vi "Patrick Builder.vi"() -> ()   [LabVIEW 2019]
uses:
  VIPM/Typedefs/File Type--enum.ctl
  <vilib>/Utility/sysdir.llb/System Directory Type.ctl
  <vilib>/Hampel Software Engineering/Git API/Git API/GIT-api.lvclass
  <vilib>/Utility/file.llb/Read Delimited Spreadsheet (string).vi
  <vilib>/Utility/file.llb/Write Delimited Spreadsheet (string).vi
  <vilib>/JKI/VIPM API/VIPM API_vipm_api.lvlib
  VIPM/VIPM.lvclass
  Git/Git.lvclass
panel:
  out "repository path":path
  out "Latest EXE":path
  out "Latest VIP":path
  in  "Mode":T1
  in  "Create File List":bool
  out "Package Builder":string
  in  "Clear Notes":bool
  in  "Release Notes":string
  in  "Append Notes":bool
  in  "ALL":bool
  in  "Patch +1":bool
  out "Selected File List":string
  in  "Publish":bool
  in  "Open List":bool
  in  "Build":bool
  in  "Preview":bool
  out "Status":string
  in  "File List":i32(listbox)
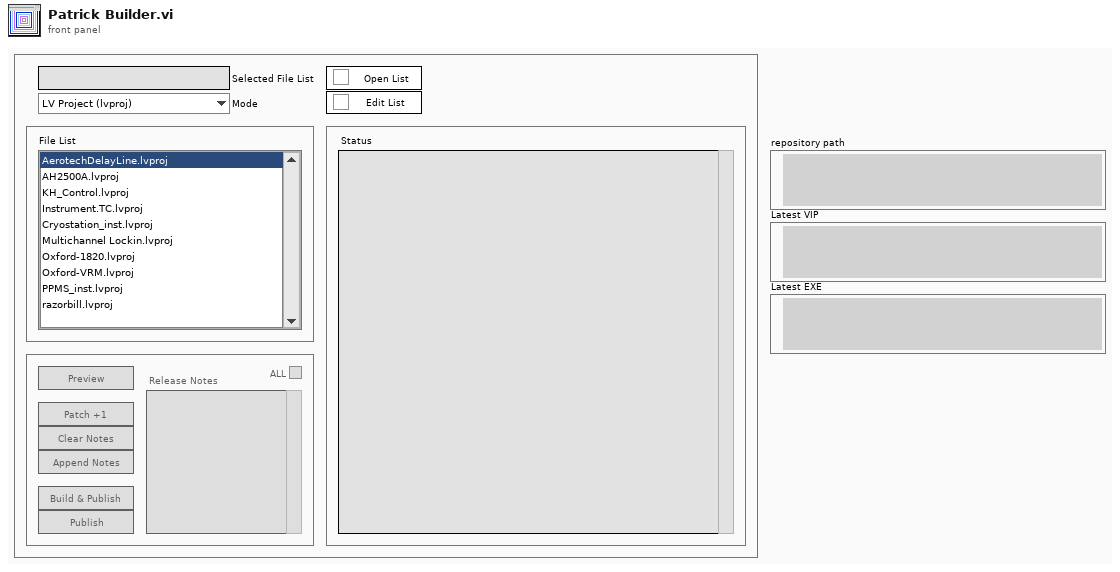
[diagram p1: front panel]
types:
  T1 = typedef "VIPM.lvclass/File Type--enum.ctl" = enum16{"LV Project (lvproj)", "Build Spec (vipb)", "Package (vip)"}
  T2 = enum32{"Invalid", "Standard", "Closed", "Hidden", "Minimized", "Maximized"}
  T3 = enum32{"invalid app kind", "Development System", "Run Time System", "Student Edition", "Embedded LabVIEW", "Evaluation", "Custom"}
  T4 = enum8{"Enabled", "Disabled", "Disabled and Grayed Out"}
  T5 = cluster{"Core":cluster{"Current VI Reference":refnum<vi>, "Close Panel on Exit?":bool}, "lvproj paths":path[], "vipb paths":path[], "vip paths":path[], "selected path":path, "config path":path, "Mode":T1, "git-api":refnum<class "GIT-api.lvclass">}
  T6 = typedef "System Directory Type.ctl" = i32
  T7 = cluster{"Current VI Reference":refnum<vi>, "Close Panel on Exit?":bool}
  T8 = typedef "VIPM API_vipm_api.lvlib/VI Package Build Spec Data Cluster_vipm_api.ctl" = cluster{"Package Version":T9, "Product Name":string, "Company Name":string, "Author Name (Person or Company)":string, "Product Homepage (URL)":string, "Legal Copyright":string, "License Agreement Name":string, "Product Description Summary":string, "Product Description":string, "Release Notes - Change Log":string}
  T9 = typedef "VIPM API_vipm_api.lvlib/Version Info Cluster_vipm_api.ctl" = cluster{"major":u32, "minor":u32, "patch":u32, "build":u32}
  T10 = typedef "VIPM API_vipm_api.lvlib/Repository Info Cluster_vipm_api.ctl" = cluster{"Repository Name":string, "Repository Folder Location":path}
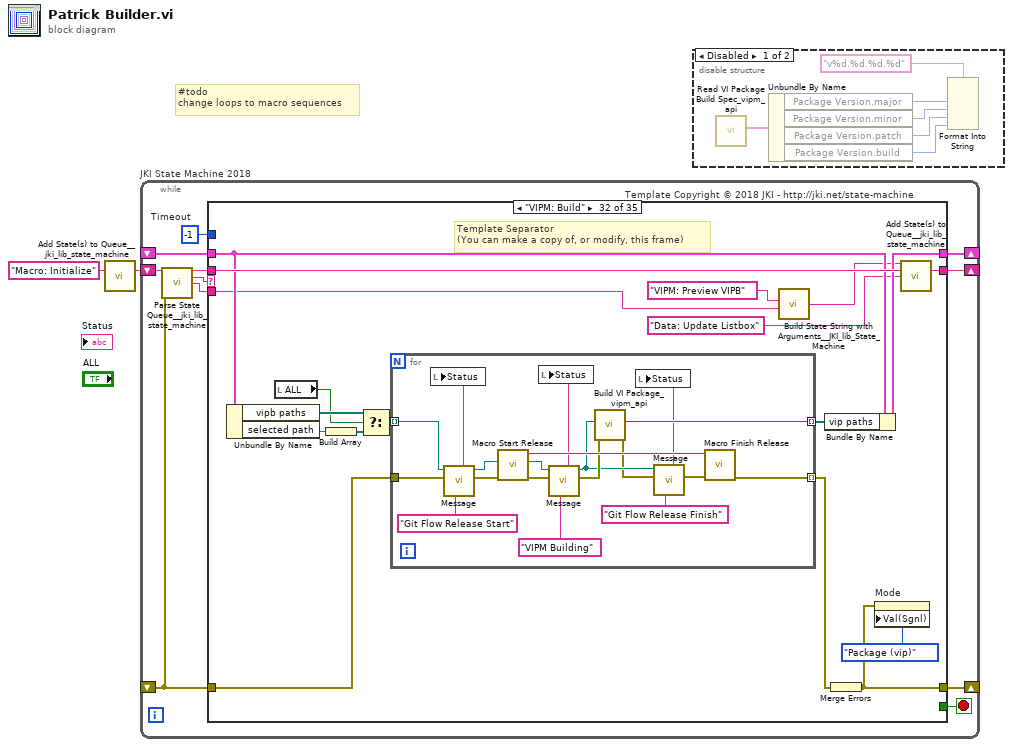
[diagram p0: block diagram]
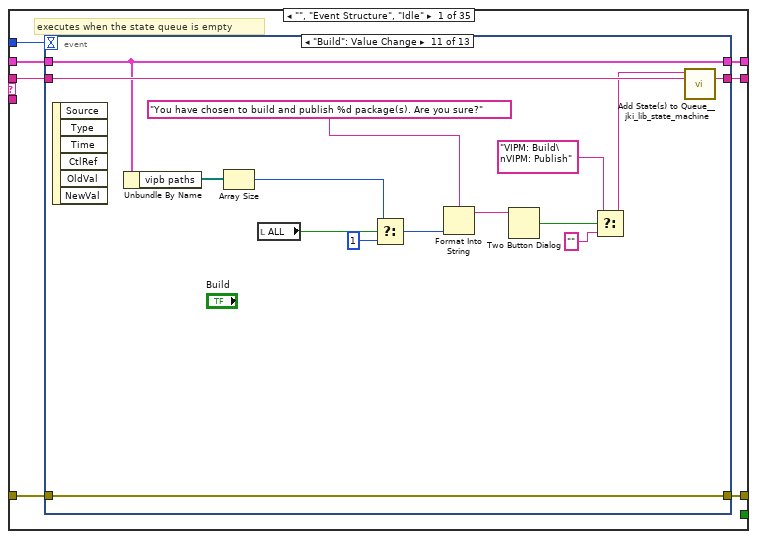
[diagram p3: hidden frame]
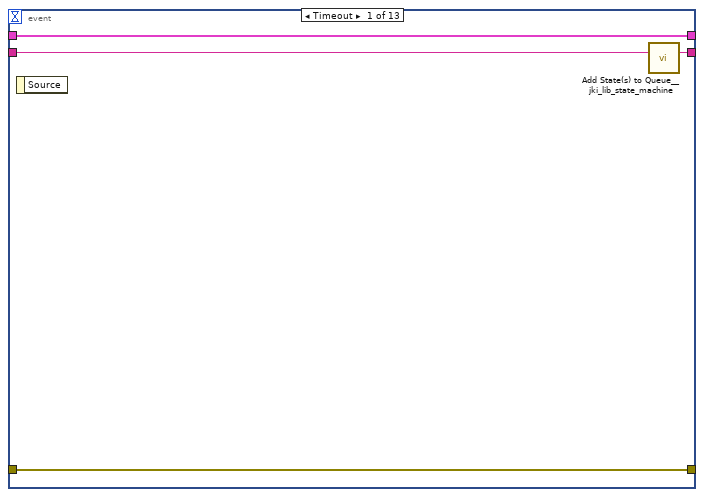
[diagram p4: hidden frame]
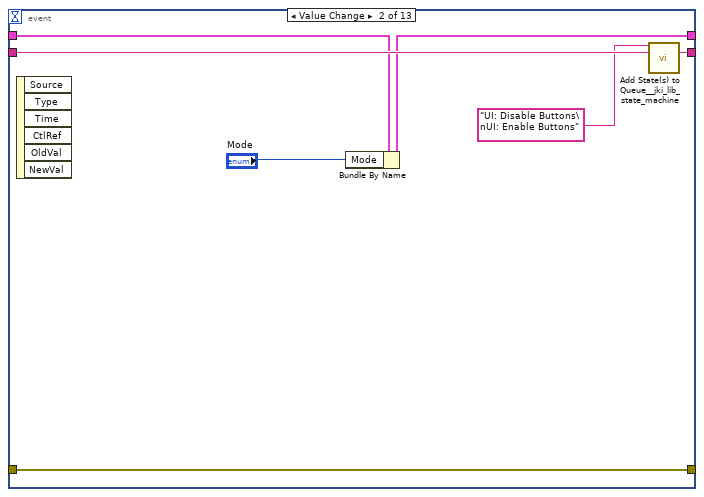
[diagram p5: hidden frame]
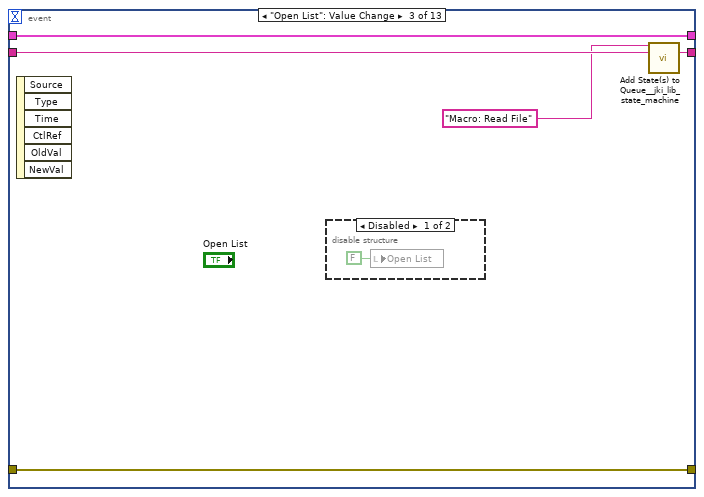
[diagram p6: hidden frame]
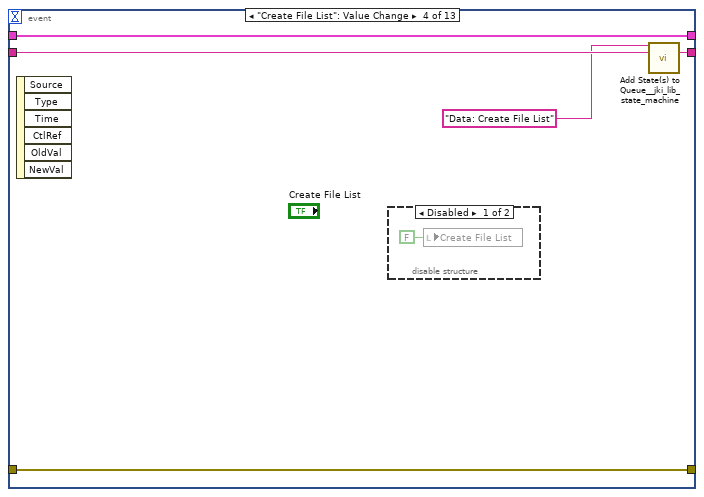
[diagram p8: hidden frame]
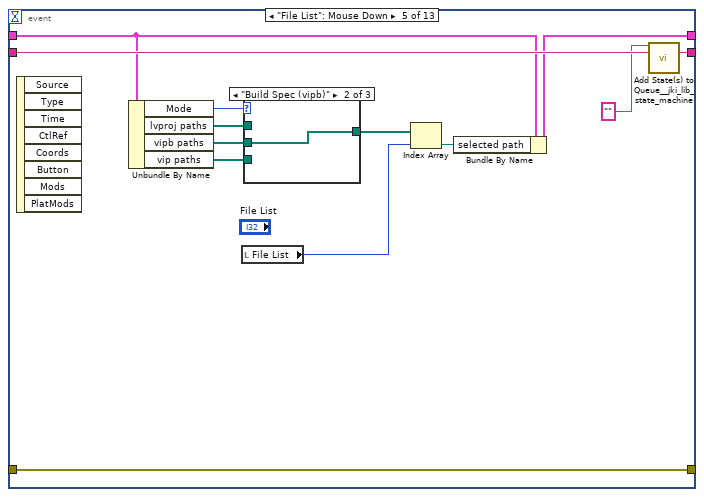
[diagram p10: hidden frame]
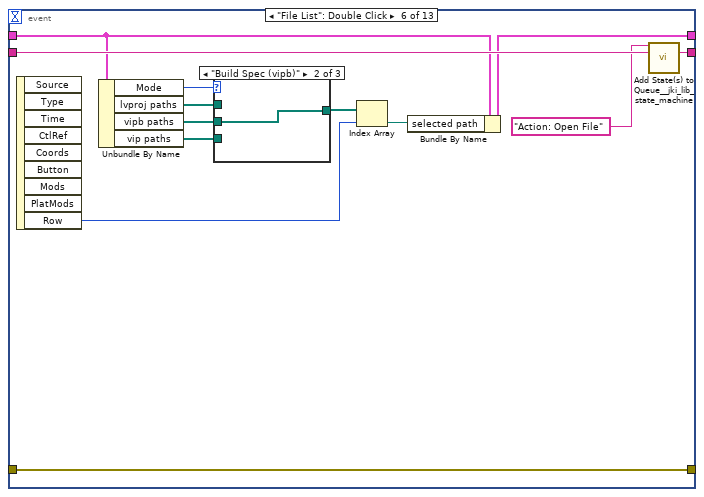
[diagram p13: hidden frame]
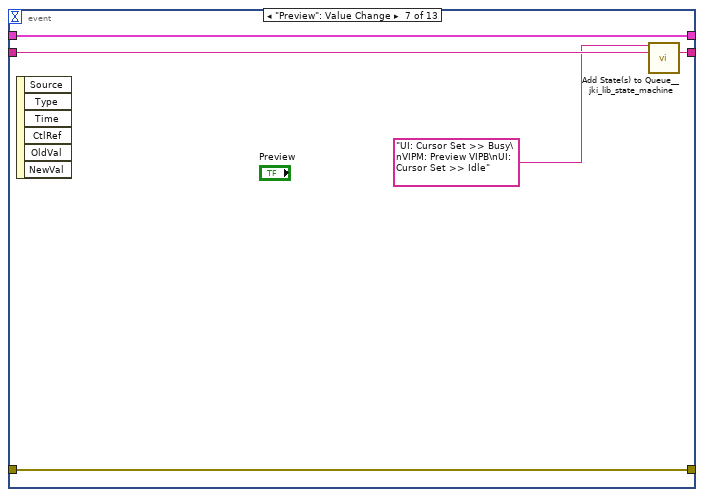
[diagram p16: hidden frame]
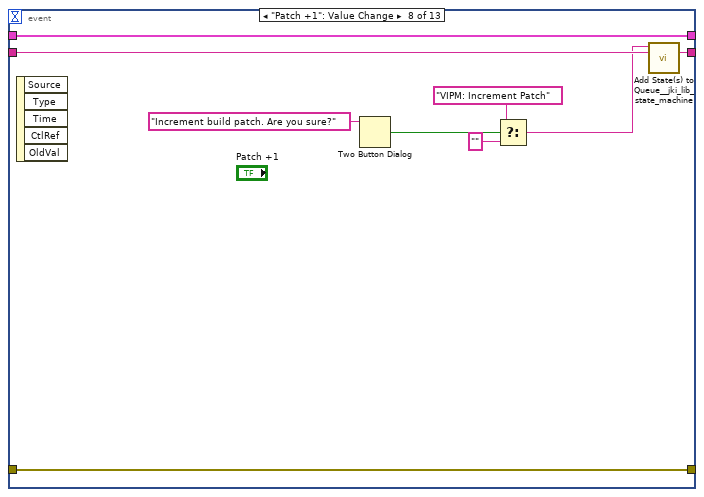
[diagram p17: hidden frame]
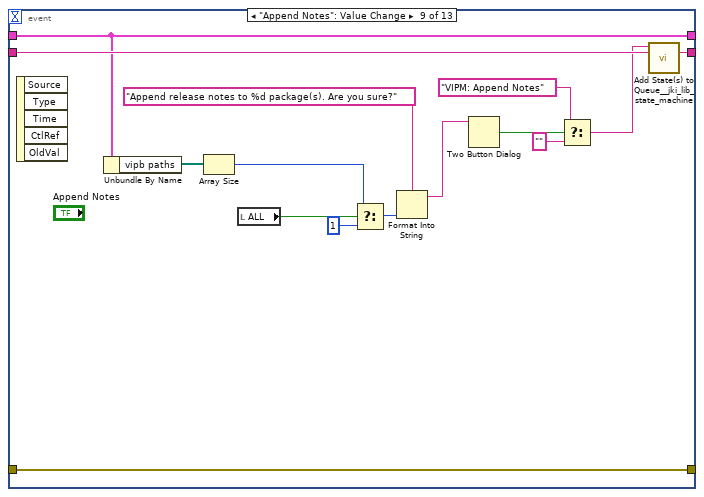
[diagram p18: hidden frame]
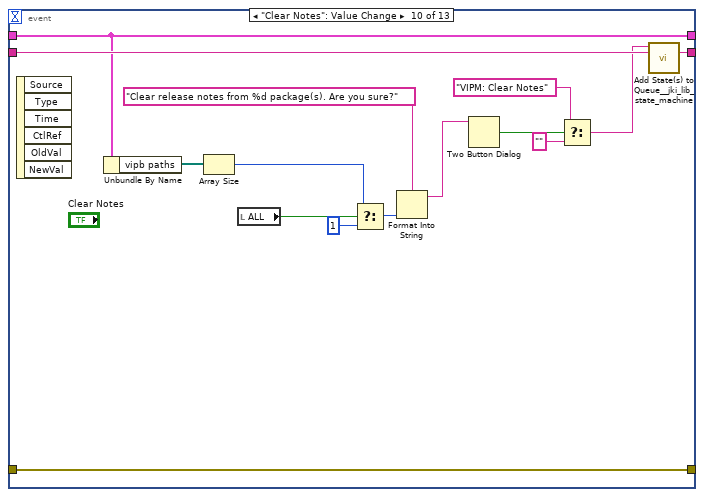
[diagram p19: hidden frame]
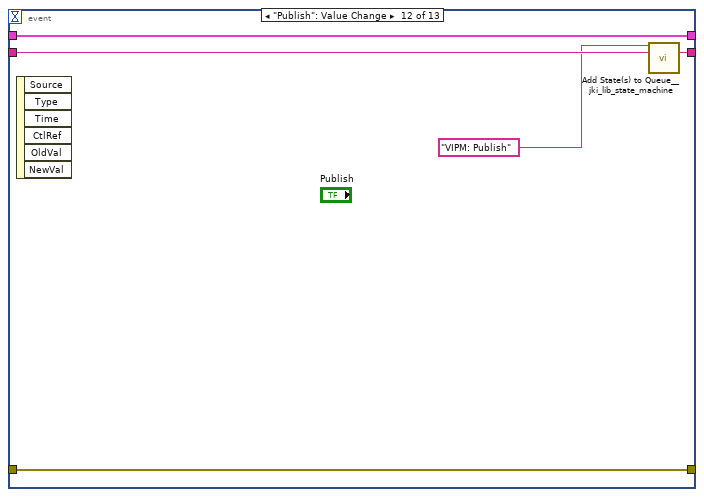
[diagram p20: hidden frame]
diagram:
  # "#todo\nchange loops to macro sequences"
  n1 = call <vilib>:"Add State(s) to Queue__jki_lib_state_machine.vi"("State(s) in (\"\")"="Macro: Initialize") -> ("States Out"=w2:string)  [unwired: 14 in]
  n2 = while "JKI State Machine 2018" {
    shift-right: [w6] -> _
    shift-left: _ -> [w5]
    shift-right: [w9] -> _
    shift-left: _ -> [w3]
    shift-right: [w8] -> _
    shift-left: w2 -> [w10]
    stop <- w7 stop-if-true
    w4 = -1  # Timeout
    # "Template Copyright © 2018 JKI - http://jki.net/state-machine"
    n3 = call <vilib>:"Parse State Queue__jki_lib_state_machine.vi"("State Queue"=w10, "Error In (no error)"=w3) -> ("Remaining States"=w12:string, "Current State"=w13:string, "Arguments"=w11:string)  [unwired: 11 in]
    n4 = case shown="\"VIPM: Build\"" w13 {
      selector: w13 -> [_ _ w150 _ _ _ _ _ _ _ _ _ _ _ _ _ _ _ _ _ _ _ _ _ _ _ _ _ _ _ _ _ _ _ _]
      tunnel: w12 -> [w20 w149 w154 w173 w180 w189 w193 w214 w220 w230 w250 w267 w300 w333 w337 w347 w360 w378 w391 w402 w471 w476 w481 w491 w495 w508 w512 w525 w545 w565 w584 w610 w642 w646 w651]
      tunnel: w11 -> [_ _ _ _ _ _ _ _ _ _ _ _ _ _ _ _ _ _ w386 w396 _ _ _ _ _ _ _ _ _ _ _ w598 _ _ _]
      tunnel: w5 -> [w18 w146 w152 w166 w177 w187 w190 _ w215 w222 w243 w259 w289 w331 w334 w345 w357 w373 w389 w398 w468 w473 w478 w488 w492 w506 w509 w523 w543 w563 w582 w603 w636 w643 w649]
      tunnel: [w17 w147 w156 w170 errorcluster {"status"=FALSE, "code"=0, "source"=""} ("error out") w186 w191 w206 w216 w228 w240 w264 w290 w327 w335 w344 w358 w376 w387 w399 w469 w474 w479 w489 w493 w501 w510 w514 w535 w554 w575 w594 w634 w644 w648] -> w9
      tunnel: w3 -> [w16 w147 w155 w170 w175 w186 w191 w205 w217 w228 w245 w265 w297 w328 w335 w343 w358 w376 w388 w400 w469 w474 w479 w489 w493 w500 w510 w522 w538 w558 w577 w596 w633 w644 w648]
      tunnel: [w19 w148 w153 w172 w179 w188 w192 w213 w219 w229 w249 w266 w299 w332 w336 w346 w359 w377 w390 w401 w470 w475 w480 w490 w494 w507 w511 w524 w544 w564 w583 w609 w641 w645 w650] -> w8
      tunnel: [_ _ _ _ _ TRUE _ _ _ _ _ _ _ _ _ _ _ _ _ _ _ _ _ _ _ _ _ _ _ _ _ _ _ _ _] -> w7
      tunnel: [w15 w146 w152 w171 w177 w187 w190 w212 w215 w226 w244 w263 w288 w331 w334 w345 w357 w373 w389 w398 w468 w473 w478 w488 w492 w506 w509 w523 w543 w563 w582 w604 w636 w643 w649] -> w6
      tunnel: w4 -> [w14 _ _ _ _ _ _ _ _ _ _ _ _ _ _ _ _ _ _ _ _ _ _ _ _ _ _ _ _ _ _ _ _ _ _]
      frame "", "Event Structure", "Idle" {
        # "executes when the state queue is empty"
        n5 = event shown="[10] \"Build\": Value Change" {
          selector: _ -> [_ _ _ _ _ _ _ _ _ _ _ _ _]
          dyn-events: _ -> [_ _ _ _ _ _ _ _ _ _ _ _ _]
          timeout: w14 -> [_ _ _ _ _ _ _ _ _ _ _ _ _]
          tunnel: w20 -> [w24 w31 w36 w42 w56 w72 w80 w89 w104 w119 w134 w139 w145]
          tunnel: [w23 w30 w35 w41 w55 w71 w79 w88 w103 w118 w133 w138 w144] -> w19
          tunnel: w18 -> [w21 w27 w32 w38 w53 w61 w77 w86 w90 w105 w127 w136 w142]
          tunnel: [w22 w29 w33 w39 w54 w70 w78 w87 w102 w117 w132 w137 w143] -> w17
          tunnel: w16 -> [w22 w29 w33 w39 w54 w70 w78 w87 w102 w117 w132 w137 w143]
          tunnel: [w21 w28 w32 w38 w52 w69 w77 w86 w90 w105 w127 w136 w142] -> w15
          event Timeout {
            n6 = event-data() -> ()  [unwired: 1 in, 1 out]
            n7 = call <vilib>:"Add State(s) to Queue__jki_lib_state_machine.vi"("State(s) in (\"\")"=w24) -> ("States Out"=w23:string)  [unwired: 14 in]
          }
          event Value Change {
            n8 = event-data() -> ()  [unwired: 1 in, 6 out]
            n9 = Bundle By Name(cluster=w27, "Mode"="Mode") -> (w28:T5)
            n10 = call <vilib>:"Add State(s) to Queue__jki_lib_state_machine.vi"("State(s) in Front (\"\")"="UI: Disable Buttons\nUI: Enable Buttons" ("State(s) in Front (\"\")"), "State(s) in (\"\")"=w31) -> ("States Out"=w30:string)  [unwired: 13 in]
          }
          event "Open List": Value Change {
            n11 = event-data() -> ()  [unwired: 1 in, 6 out]
            n12 = disable-structure shown="Disabled" {
              frame Disabled {
                n13 = local write "Open List"(FALSE ("Open List")) -> ()
              }
              frame Enabled {
              }
            }
            n14 = call <vilib>:"Add State(s) to Queue__jki_lib_state_machine.vi"("State(s) in Front (\"\")"="Macro: Read File" ("State(s) in Front (\"\")"), "State(s) in (\"\")"=w36) -> ("States Out"=w35:string)  [unwired: 13 in]
          }
          event "Create File List": Value Change {
            n15 = event-data() -> ()  [unwired: 1 in, 6 out]
            n16 = disable-structure shown="Disabled" {
              frame Disabled {
                n17 = local write "Create File List"(FALSE ("Create File List")) -> ()
              }
              frame Enabled {
              }
            }
            n18 = call <vilib>:"Add State(s) to Queue__jki_lib_state_machine.vi"("State(s) in Front (\"\")"="Data: Create File List" ("State(s) in Front (\"\")"), "State(s) in (\"\")"=w42) -> ("States Out"=w41:string)  [unwired: 13 in]
          }
          event "File List": Mouse Down {
            n19 = event-data() -> ()  [unwired: 1 in, 8 out]
            n20 = Unbundle By Name(w53) -> ("Mode"=w48:T1, "lvproj paths"=w45:path[], "vipb paths"=w44:path[], "vip paths"=w46:path[])
            n21 = local read "File List"() -> (w49:i32)
            n22 = case shown="\"Build Spec (vipb)\"" w48 {
              tunnel: [w57 w58 w59] -> w47
              tunnel: w46 -> [_ _ w59]
              tunnel: w45 -> [w57 _ _]
              tunnel: w44 -> [_ w58 _]
              frame "LV Project (lvproj)", Default {
              }
              frame "Build Spec (vipb)" {
              }
              frame "Package (vip)" {
              }
            }
            n23 = Index Array(array=w47, index=w49) -> (element=w51:path)
            n24 = Bundle By Name(cluster=w53, "selected path"=w51) -> (w52:T5)
            n25 = call <vilib>:"Add State(s) to Queue__jki_lib_state_machine.vi"("State(s) in Front (\"\")"="" ("State(s) in Front (\"\")"), "State(s) in (\"\")"=w56) -> ("States Out"=w55:string)  [unwired: 13 in]
          }
          event "File List": Double Click {
            n26 = event-data() -> ("Row"=w66:i32)  [unwired: 1 in, 8 out]
            n27 = Unbundle By Name(w61) -> ("Mode"=w65:T1, "lvproj paths"=w63:path[], "vipb paths"=w62:path[], "vip paths"=w64:path[])
            n28 = case shown="\"Build Spec (vipb)\"" w65 {
              tunnel: [w73 w74 w75] -> w60
              tunnel: w64 -> [_ _ w75]
              tunnel: w63 -> [w73 _ _]
              tunnel: w62 -> [_ w74 _]
              frame "LV Project (lvproj)", Default {
              }
              frame "Build Spec (vipb)" {
              }
              frame "Package (vip)" {
              }
            }
            n29 = Index Array(array=w60, index=w66) -> (element=w68:path)
            n30 = Bundle By Name(cluster=w61, "selected path"=w68) -> (w69:T5)
            n31 = call <vilib>:"Add State(s) to Queue__jki_lib_state_machine.vi"("State(s) in Front (\"\")"="Action: Open File" ("State(s) in Front (\"\")"), "State(s) in (\"\")"=w72) -> ("States Out"=w71:string)  [unwired: 13 in]
          }
          event "Preview": Value Change {
            n32 = event-data() -> ()  [unwired: 1 in, 6 out]
            n33 = call <vilib>:"Add State(s) to Queue__jki_lib_state_machine.vi"("State(s) in Front (\"\")"="UI: Cursor Set >> Busy\nVIPM: Preview VIPB\nUI: Cursor Set >> Idle" ("State(s) in Front (\"\")"), "State(s) in (\"\")"=w80) -> ("States Out"=w79:string)  [unwired: 13 in]
          }
          event "Patch +1": Value Change {
            n34 = event-data() -> ()  [unwired: 1 in, 5 out]
            n35 = Two Button Dialog(message="Increment build patch. Are you sure?") -> (T button?=w84:bool)  [unwired: 2 in]
            n36 = Select(t="VIPM: Increment Patch" ("State(s) in Front (\"\")"), s=w84, f="") -> (s? t:f=w81:string)
            n37 = call <vilib>:"Add State(s) to Queue__jki_lib_state_machine.vi"("State(s) in Front (\"\")"=w81, "State(s) in (\"\")"=w89) -> ("States Out"=w88:string)  [unwired: 13 in]
          }
          event "Append Notes": Value Change {
            n38 = event-data() -> ()  [unwired: 1 in, 5 out]
            n39 = Unbundle By Name(w90) -> ("vipb paths"=w97:path[])
            n40 = Array Size(array=w97) -> (size(s)=w95:i32)
            n41 = local read "ALL"() -> (w96:bool)
            n42 = Select(t=w95, s=w96, f=1) -> (s? t:f=w98:i32)
            n43 = Format Into String(format string="Append release notes to %d package(s). Are you sure?" ("message"), w98) -> (resulting string=w92:string)  [unwired: 2 in, 1 out]
            n44 = Two Button Dialog(message=w92) -> (T button?=w101:bool)  [unwired: 2 in]
            n45 = Select(t="VIPM: Append Notes" ("State(s) in Front (\"\")"), s=w101, f="") -> (s? t:f=w99:string)
            n46 = call <vilib>:"Add State(s) to Queue__jki_lib_state_machine.vi"("State(s) in Front (\"\")"=w99, "State(s) in (\"\")"=w104) -> ("States Out"=w103:string)  [unwired: 13 in]
          }
          event "Clear Notes": Value Change {
            n47 = event-data() -> ()  [unwired: 1 in, 6 out]
            n48 = Unbundle By Name(w105) -> ("vipb paths"=w112:path[])
            n49 = Array Size(array=w112) -> (size(s)=w110:i32)
            n50 = local read "ALL"() -> (w111:bool)
            n51 = Select(t=w110, s=w111, f=1) -> (s? t:f=w113:i32)
            n52 = Format Into String(format string="Clear release notes from %d package(s). Are you sure?" ("message"), w113) -> (resulting string=w107:string)  [unwired: 2 in, 1 out]
            n53 = Two Button Dialog(message=w107) -> (T button?=w116:bool)  [unwired: 2 in]
            n54 = Select(t="VIPM: Clear Notes" ("State(s) in Front (\"\")"), s=w116, f="") -> (s? t:f=w114:string)
            n55 = call <vilib>:"Add State(s) to Queue__jki_lib_state_machine.vi"("State(s) in Front (\"\")"=w114, "State(s) in (\"\")"=w119) -> ("States Out"=w118:string)  [unwired: 13 in]
          }
          event "Build": Value Change {
            n56 = event-data() -> ()  [unwired: 1 in, 6 out]
            n57 = Unbundle By Name(w127) -> ("vipb paths"=w126:path[])
            n58 = Array Size(array=w126) -> (size(s)=w124:i32)
            n59 = local read "ALL"() -> (w125:bool)
            n60 = Select(t=w124, s=w125, f=1) -> (s? t:f=w122:i32)
            n61 = Format Into String(format string="You have chosen to build and publish %d package(s). Are you sure?" ("message"), w122) -> (resulting string=w121:string)  [unwired: 2 in, 1 out]
            n62 = Two Button Dialog(message=w121) -> (T button?=w131:bool)  [unwired: 2 in]
            n63 = Select(t="VIPM: Build\nVIPM: Publish" ("State(s) in Front (\"\")"), s=w131, f="") -> (s? t:f=w128:string)
            n64 = call <vilib>:"Add State(s) to Queue__jki_lib_state_machine.vi"("State(s) in Front (\"\")"=w128, "State(s) in (\"\")"=w134) -> ("States Out"=w133:string)  [unwired: 13 in]
          }
          event "Publish": Value Change {
            n65 = event-data() -> ()  [unwired: 1 in, 6 out]
            n66 = call <vilib>:"Add State(s) to Queue__jki_lib_state_machine.vi"("State(s) in Front (\"\")"="VIPM: Publish" ("State(s) in Front (\"\")"), "State(s) in (\"\")"=w139) -> ("States Out"=w138:string)  [unwired: 13 in]
          }
          event Panel Close? {
            # "Discard the event because we'll close the front panel ourselves in Macro: Exit"
            # "Close Panel button (pressed) Event\n(this executes Macro: Exit to terminate the VI)"
            n67 = event-data() -> ()  [unwired: 1 in, 1 out]
            n68 = event-data("Discard?"=TRUE) -> ()  [unwired: 1 in, 1 out]
            n69 = call <vilib>:"Add State(s) to Queue__jki_lib_state_machine.vi"("State(s) in Front (\"\")"="Macro: Exit", "State(s) in (\"\")"=w145) -> ("States Out"=w144:string)  [unwired: 13 in]
          }
        }
      }
      frame "---------- Core ----------" {
        # "Do not put any code in this frame.\n(it is a separator no-op)"
        n70 = call <vilib>:"Add State(s) to Queue__jki_lib_state_machine.vi"("State(s) in (\"\")"=w149) -> ("States Out"=w148:string)  [unwired: 14 in]
      }
      frame Default {
        w159 = 42 items=["No error", "Argument error", "Memory is full", "Out of zone", "End of file", "File already open", "Generic file I/O error", "File not found", "File permission error", "Disk is full", "Duplicate path", "Too many files open", "System feature not enabled", "Resource file not found", "Cannot add resource", "Resource not found", "Image not found", "Image memory error", "Pen does not exist", "Config type invalid", "Config token not found", "Config parse error", "Config memory error", "Bad external code format", "Bad external code offset", "External code not present", "Null window", "Destroy window error", "Null menu", "Print aborted", "Bad print record", "Print driver error", "Windows error during printing", "Memory error during printing", "Print dialog error", "Generic print error", "Invalid device refnum", "Device not found", "Device parameter error", "Device unit error", "Cannot open device", "Device call aborted", "Generic error", "Cancelled by user", "Object ID too low", "Object ID too high", "Object not in heap", "Unknown heap", "Unknown object (invalid DefProc)", "Unknown object (DefProc not in table)", "Message out of range", "Invalid (null) method", "Unknown message", "Manager call not supported", "Bad address", "Network operation in progress", "Network operation timed out", "Connection is busy", "Network attribute not supported", "Network error", "Address in use", "System out of memory", "Connection aborted", "Connection refused", "Not connected", "Already connected", "Connection closed", "Initialization error (interapplication manager)", "Bad occurrence", "Wait on unbound occurrence handler", "Occurrence queue overflow", "Datalog type conflict", "Unused", "Unrecognized type (interapplication manager)", "Memory corrupt", "Failed to make temporary DLL", "Old CIN version", "Drag socket not found", "Failed to load drop-object", "Failed to register OLE object", "Failed to release OLE object", "Format specifier type mismatch", "Unknown format specifier", "Too few format specifiers", "Too many format specifiers", "Scan failed", "Newer CIN version", "Error converting to variant", "Runtime menu error", "Password tampered", "Variant attribute not found", "Incompatible variant data type", "Event data is not available", "Event Store is not present", "Occurrence is not found", "Event Queue is not created", "Event info is not available", "Refnum passed is NULL", "Error retrieving Class GUID", "Error retrieving CoClass GUID", "Error retrieving TypeLib GUID.", "Bad built application magic bytes.", "Specific driver is different from the specific driver associated with the Logical Name.", "There is no session opened to the class driver.", "Max Error", "MAX - Error with config objects", "MAX - Error loading configuration", "MAX - Group not supported"]
        # "Current State"
        # "Do not delete, rename, or modify this frame.\n(this is used to capture unhandled states and typos)"
        # "Handle mistyped state name (developer tool)"
        n71 = Format Into String(format string="Software Exception: Unhandled State \"%s\"." ("message"), error in=w155, w150) -> (resulting string=w158:string, error out=w157:errorcluster)  [unwired: 1 in]
        n72 = call <vilib>:"Error Cluster From Error Code.vi"("show call chain? (False)"=TRUE, "error in (no error)"=w157, "error message (\"\")"=w158, "error code (0)"=w159) -> ("error out"=w156:errorcluster)  [unwired: 5 in]
        n73 = call <vilib>:"Add State(s) to Queue__jki_lib_state_machine.vi"("State(s) in (\"\")"=w154) -> ("States Out"=w153:string)  [unwired: 14 in]
      }
      frame "Initialize Core Data" {
        # "Do not delete, rename, or modify this frame.\n(this is used to determine panel behavior on exit)"
        # "originally closed?"
        # "exe?"
        # "If panel starts closed or is an EXE, then close it when we exit"
        n74 = property class="VI"() -> ("FP.State"=w163:T2)  [unwired: 2 in, 2 out]
        n75 = property class="App"() -> ("App.Kind"=w169:T3)  [unwired: 2 in, 2 out]
        n76 = control-ref of="Current VI Reference"() -> (w164:refnum<vi>)
        n77 = Equal?(x=w163, y=T2."Closed" ("Front Panel Window:State")) -> (x = y?=w161:bool)
        n78 = Equal?(x=w169, y=T3."Run Time System" ("Application:Kind")) -> (x = y?=w167:bool)
        n79 = Or(x=w161, y=w167) -> (x .or. y?=w165:bool)
        n80 = Bundle By Name(cluster=w166, "Core.Current VI Reference"=w164, "Core.Close Panel on Exit?"=w165) -> (w171:T5)
        n81 = call <vilib>:"Add State(s) to Queue__jki_lib_state_machine.vi"("State(s) in (\"\")"=w173) -> ("States Out"=w172:string)  [unwired: 14 in]
      }
      frame "Error Handler" {
        # "Unhandled Error -- Display it"
        # "Handle any errors here.\nYou can also output any states to clean-up after errors occur"
        # "Clear error"
        n82 = case shown="Error 1059" w175 {
          selector: w175 -> [w181 w182 _]
          tunnel: [w181 w182 w183] -> w174
          frame No Error {
          }
          frame Default {
          }
          frame Error {
            n83 = property on="Open List" class="Bool"("Val(Sgnl)"=TRUE) -> (error out=w183:errorcluster)  [unwired: 2 in, 1 out]
          }
        }
        n84 = call <vilib>:"General Error Handler.vi"("error in (no error)"=w174) -> ()  [unwired: 10 in, 5 out]
        n85 = call <vilib>:"Add State(s) to Queue__jki_lib_state_machine.vi"("State(s) in Front (\"\")"="/* Post Error States", "State(s) in (\"\")"=w180) -> ("States Out"=w179:string)  [unwired: 13 in]
      }
      frame "Exit" {
        # "Do not put any code in this frame.\n(No errors that occur here will be handled.)"
        n86 = call <vilib>:"Add State(s) to Queue__jki_lib_state_machine.vi"("State(s) in (\"\")"=w189) -> ("States Out"=w188:string)  [unwired: 14 in]
      }
      frame "---------- Data ----------" {
        # "Do not put any code in this frame.\n(It is a separator no-op. You can make a copy of this frame to create a new Data frame)"
        n87 = call <vilib>:"Add State(s) to Queue__jki_lib_state_machine.vi"("State(s) in (\"\")"=w193) -> ("States Out"=w192:string)  [unwired: 14 in]
      }
      frame "Data: Initialize" {
        w194 = refnum<class "GIT-api.lvclass"> refnum  # git-api
        w195 = File_Type--enum."LV Project (lvproj)"  # Mode
        w201 = T6 3 items=["User Home"=0, "User Desktop"=1, "User Documents"=2, "User Application Data"=3, "User Preferences"=4, "User Temporary"=5, "Public Documents"=6, "Public Application Data"=7, "Public Preferences"=8, "Public Cache"=13, "System Core Libraries"=9, "System Installed Libraries"=10, "Application Files"=11, "Boot Volume Root"=12] ("system directory type")
        w202 = path[] []  # lvproj paths
        w203 = path[] []  # vip paths
        w204 = path[] []  # vipb paths
        w208 = path ""  # config path
        w210 = path ""  # selected path
        w211 = T7 {"Current VI Reference"=refnum, "Close Panel on Exit?"=FALSE}  # Core
        # "Initialize the shift-register data, here.\n(data names are defined by what you wire into the bundle function)"
        n88 = call <vilib>:"Get System Directory.vi"("system directory type"=w201) -> ("system directory"=w198:path)  [unwired: 10 in]
        n89 = Build Path(base path=w198, name or relative path="LevyLab") -> (appended path=w197:path)
        n90 = Build Path(base path=w197, name or relative path="build-support") -> (appended path=w199:path)
        n91 = call <userlib>:"Create Dir if Non-Existant__ogtk.vi"("error in (no error)"=w205, "Directory Path"=w199) -> ("error out"=w206:errorcluster, "dup Directory Path"=w207:path)  [unwired: 7 in, 1 out]
        n92 = Variant To Data(type=w208, Variant=w207) -> (data=w209:path)  [unwired: 1 in, 1 out]
        n93 = Bundle("Core"=w211, "lvproj paths"=w202, "vipb paths"=w204, "vip paths"=w203, "selected path"=w210, "config path"=w209, "Mode"=w195, "git-api"=w194) -> (w212:T5)  [unwired: 1 in]
        n94 = call <vilib>:"Add State(s) to Queue__jki_lib_state_machine.vi"("State(s) in (\"\")"=w214) -> ("States Out"=w213:string)  [unwired: 14 in]
      }
      frame "Data: Cleanup" {
        # "Cleanup any data and references, here.\n(this is called automatically, by the Macro: Exit)"
        n95 = Unbundle By Name(w215) -> ("Core.Current VI Reference"=w218:refnum<vi>)
        n96 = Close Reference(reference=w218, error in (no error)=w217) -> (error out=w216:errorcluster)
        n97 = call <vilib>:"Add State(s) to Queue__jki_lib_state_machine.vi"("State(s) in (\"\")"=w220) -> ("States Out"=w219:string)  [unwired: 14 in]
      }
      frame "Data: Update Listbox" {
        w224 = 0 ("Value (Signaling)")
        # "Do not put any code in this frame.\n(It is a separator no-op. You can make a copy of this frame to create a new Data frame)"
        n98 = Unbundle By Name(w222) -> ("Mode"=w223:T1)
        n99 = case shown="\"Package (vip)\"" w223 {
          tunnel: w222 -> [w232 w234 w236]
          tunnel: [w231 w233 w235] -> w221
          frame "LV Project (lvproj)", Default {
            n100 = Unbundle By Name(w232) -> ("lvproj paths"=w231:path[])
          }
          frame "Build Spec (vipb)" {
            n101 = Unbundle By Name(w234) -> ("vipb paths"=w233:path[])
          }
          frame "Package (vip)" {
            n102 = Unbundle By Name(w236) -> ("vip paths"=w235:path[])
          }
        }
        n103 = for {
          tunnel: w221 -> [w238] mode=indexing
          tunnel: [w237] -> w227 mode=indexing
          n104 = Strip Path(path=w238) -> (name=w237:string)  [unwired: 1 out]
        }
        n105 = property on="File List" class="LstBox (strict)"("Item Names"=w227, "Val(Sgnl)"=w224) -> ()  [unwired: 2 in, 2 out]
        n106 = Index Array(array=w221, index=w224) -> (element=w225:path)
        n107 = Bundle By Name(cluster=w222, "selected path"=w225) -> (w226:T5)
        n108 = call <vilib>:"Add State(s) to Queue__jki_lib_state_machine.vi"("State(s) in (\"\")"=w230) -> ("States Out"=w229:string)  [unwired: 14 in]
      }
      frame "Data: Choose File List" {
        # "Do not put any code in this frame.\n(It is a separator no-op. You can make a copy of this frame to create a new Data frame)"
        n109 = Unbundle By Name(w243) -> ("config path"=w248:path)
        n110 = call "File Dialog"("start path"=w248, "error in"=w245, "pattern (all files)"="*.txt") -> ("selected path"=w247:path, "cancelled"=w242:bool, "error out"=w241:errorcluster)  [unwired: 9 in, 1 out]
        n111 = case shown="False" w242 {
          tunnel: w247 -> [w251 _]
          tunnel: [w255 _] -> w246
          tunnel: [w254 w256] -> w244
          tunnel: w243 -> [w253 w256]
          tunnel: w241 -> [w252 _]
          tunnel: [w252 _] -> w240
          frame False {
            n112 = Bundle By Name(cluster=w253, "config path"=w251) -> (w254:T5)
            n113 = Strip Path(path=w251) -> (name=w255:string)  [unwired: 1 out]
          }
          frame True {
          }
        }
        "Selected File List" <- w246
        n114 = call <vilib>:"Add State(s) to Queue__jki_lib_state_machine.vi"("State(s) in (\"\")"=w250) -> ("States Out"=w249:string)  [unwired: 14 in]
      }
      frame "Data: Create File List" {
        # "Do not put any code in this frame.\n(It is a separator no-op. You can make a copy of this frame to create a new Data frame)"
        n115 = Unbundle By Name(w259) -> ("config path"=w258:path, "Mode"=w257:T1)
        n116 = call "Build File List Window.vi"("error in"=w265, "File Type"=w257, "Path"=w258) -> ("error out"=w264:errorcluster, "File Type out"=w262:T1, "files out"=w261:path[])  [unwired: 6 in]
        n117 = Empty Array?(array=w261) -> (empty?=w260:bool)
        n118 = case shown="False" w260 {
          tunnel: [w271 w284] -> w263
          tunnel: w259 -> [w270 w284]
          tunnel: w262 -> [w269 _]
          tunnel: w261 -> [w268 _]
          frame False {
            n119 = case shown="\"Package (vip)\"" w269 {
              selector: w269 -> [w272 w276 w280]
              tunnel: [w275 w279 w283] -> w271
              tunnel: w270 -> [w274 w278 w282]
              tunnel: w268 -> [w273 w277 w281]
              frame "LV Project (lvproj)" {
                n120 = Bundle By Name(cluster=w274, "lvproj paths"=w273, "Mode"=w272) -> (w275:T5)
              }
              frame "Build Spec (vipb)" {
                n121 = Bundle By Name(cluster=w278, "vipb paths"=w277, "Mode"=w276) -> (w279:T5)
              }
              frame "Package (vip)" {
                n122 = Bundle By Name(cluster=w282, "vip paths"=w281, "Mode"=w280) -> (w283:T5)
              }
            }
          }
          frame True {
          }
        }
        n123 = call <vilib>:"Add State(s) to Queue__jki_lib_state_machine.vi"("State(s) in (\"\")"=w267) -> ("States Out"=w266:string)  [unwired: 14 in]
      }
      frame "Data: Read File List" {
        # "Do not put any code in this frame.\n(It is a separator no-op. You can make a copy of this frame to create a new Data frame)"
        n124 = Unbundle By Name(w289) -> ("config path"=w298:path)
        n125 = call-poly <vilib>:"Read Delimited Spreadsheet.vi"("file path (dialog if empty)"=w298, "error in (no error)"=w297, "transpose? (F)"=TRUE, "delimiter (\\t)"="\\n" ("delimiter (\\t)")) -> ("all rows"=w295:string[][], "error out"=w291:errorcluster)  [unwired: 6 in, 4 out]
        n126 = Index Array(array=w295) -> (element=w294:string[])  [unwired: 2 in]
        n127 = String To Path(string=w294) -> (path=w292:path[])
        n128 = for {
          tunnel: w292 -> [w323] mode=indexing
          tunnel: w291 -> [w322]
          tunnel: [w321] -> w290
          tunnel: [w319] -> w287 mode=indexing
          tunnel: [w318] -> w285
          n129 = call <vilib>:"Get File Extension.vi"("error in (no error)"=w322, "file"=w323) -> ("error out"=w321:errorcluster, "lowercase file extension"=w320:string, "dup file"=w319:path)  [unwired: 5 in, 2 out]
          n130 = call "Extension to Mode.vi"("lowercase file extension"=w320) -> ("Mode"=w318:T1)  [unwired: 10 in]
        }
        n131 = Empty Array?(array=w287) -> (empty?=w286:bool)
        n132 = case shown="False" w286 {
          tunnel: [w304 w317] -> w288
          tunnel: w289 -> [w303 w317]
          tunnel: w285 -> [w301 _]
          tunnel: w287 -> [w302 _]
          frame False {
            n133 = case shown="\"Build Spec (vipb)\"" w301 {
              selector: w301 -> [w305 w309 w313]
              tunnel: [w308 w312 w316] -> w304
              tunnel: w303 -> [w307 w311 w315]
              tunnel: w302 -> [w306 w310 w314]
              frame "LV Project (lvproj)" {
                n134 = Bundle By Name(cluster=w307, "lvproj paths"=w306, "Mode"=w305) -> (w308:T5)
              }
              frame "Build Spec (vipb)" {
                n135 = Bundle By Name(cluster=w311, "vipb paths"=w310, "Mode"=w309) -> (w312:T5)
              }
              frame "Package (vip)" {
                n136 = Bundle By Name(cluster=w315, "vip paths"=w314, "Mode"=w313) -> (w316:T5)
              }
            }
            n137 = local write "Mode"(w301) -> ()
          }
          frame True {
          }
        }
        n138 = call <vilib>:"Add State(s) to Queue__jki_lib_state_machine.vi"("State(s) in (\"\")"=w300) -> ("States Out"=w299:string)  [unwired: 14 in]
      }
      frame "Data: Save File List" {
        # "Do not put any code in this frame.\n(It is a separator no-op. You can make a copy of this frame to create a new Data frame)"
        n139 = Unbundle By Name(w331) -> ("config path"=w326:path, "vipb paths"=w330:path[])
        n140 = Path To String(path=w330) -> (string=w329:string[])
        n141 = call-poly <vilib>:"Write Delimited Spreadsheet.vi"("file path (dialog if empty)"=w326, "1D data"=w329, "error in (no error)"=w328, "transpose? (no:F)"=TRUE, "delimiter (\\t)"="\\n" ("delimiter (\\t)")) -> ("error out"=w327:errorcluster)  [unwired: 9 in, 1 out]
        n142 = call <vilib>:"Add State(s) to Queue__jki_lib_state_machine.vi"("State(s) in (\"\")"=w333) -> ("States Out"=w332:string)  [unwired: 14 in]
      }
      frame "---------- UI ----------" {
        # "Do not put any code in this frame.\n(It is a separator no-op. You can make a copy of this frame to create a new UI frame)"
        n143 = call <vilib>:"Add State(s) to Queue__jki_lib_state_machine.vi"("State(s) in (\"\")"=w337) -> ("States Out"=w336:string)  [unwired: 14 in]
      }
      frame "UI: Initialize" {
        # "Initialize the User Interface, here.\n(this is called automatically, by the Macro: Init)"
        n144 = call <userlib>:"MGI Get Executable Version.vi"() -> ("Version"=w340:string)  [unwired: 7 in]
        n145 = local write "Status"("" ("Status")) -> ()
        n146 = Format Into String(format string="Patrick Builder v%s", w340) -> (resulting string=→"Package Builder":string)  [unwired: 2 in, 1 out]
        n147 = call <userlib>:"Fit VI window to Largest Dec__ogtk.vi"("error in (no error)"=w343, "border spacing (2 px)"=0) -> ("error out"=w344:errorcluster)  [unwired: 4 in, 1 out]
        n148 = call <vilib>:"Add State(s) to Queue__jki_lib_state_machine.vi"("State(s) in (\"\")"=w347) -> ("States Out"=w346:string)  [unwired: 14 in]
      }
      frame "UI: Disable Buttons" {
        # "Do not put any code in this frame.\n(It is a separator no-op. You can make a copy of this frame to create a new UI frame)"
        n149 = control-ref of="Preview"() -> (w356:refnum<vi>)
        n150 = control-ref of="Build"() -> (w355:refnum<vi>)
        n151 = control-ref of="Publish"() -> (w353:refnum<vi>)
        n152 = control-ref of="Clear Notes"() -> (w352:refnum<vi>)
        n153 = control-ref of="Append Notes"() -> (w351:refnum<vi>)
        n154 = control-ref of="Patch +1"() -> (w350:refnum<vi>)
        n155 = control-ref of="Release Notes"() -> (w349:refnum<vi>)
        n156 = control-ref of="ALL"() -> (w348:refnum<vi>)
        n157 = Build Array(w356, w355, w353, w352, w351, w350, w349, w348) -> (w354:refnum<vi>[])
        n158 = for {
          tunnel: w354 -> [w361] mode=indexing
          n159 = property class="Ctl"(reference=w361, "DisabledEnum"=T4."Disabled and Grayed Out" ("Disabled")) -> ()  [unwired: 1 in, 2 out]
        }
        n160 = call <vilib>:"Add State(s) to Queue__jki_lib_state_machine.vi"("State(s) in (\"\")"=w360) -> ("States Out"=w359:string)  [unwired: 14 in]
      }
      frame "UI: Enable Buttons" {
        # "Do not put any code in this frame.\n(It is a separator no-op. You can make a copy of this frame to create a new UI frame)"
        n161 = Unbundle By Name(w373) -> ("Mode"=w365:T1, "vipb paths"=w363:path[])
        n162 = control-ref of="Preview"() -> (w375:refnum<vi>)
        n163 = control-ref of="Build"() -> (w374:refnum<vi>)
        n164 = control-ref of="Clear Notes"() -> (w372:refnum<vi>)
        n165 = control-ref of="Append Notes"() -> (w371:refnum<vi>)
        n166 = control-ref of="Patch +1"() -> (w369:refnum<vi>)
        n167 = control-ref of="Release Notes"() -> (w368:refnum<vi>)
        n168 = control-ref of="ALL"() -> (w367:refnum<vi>)
        n169 = Empty Array?(array=w363) -> (empty?=w366:bool)
        n170 = Build Array(w375, w374, w372, w371, w369, w368, w367) -> (w370:refnum<vi>[])
        n171 = Not(x=w366) -> (.not. x?=w364:bool)
        n172 = case shown="\"LV Project (lvproj)\"" w365 {
          tunnel: w370 -> [_ _ w382]
          tunnel: w364 -> [_ _ w381]
          frame "Package (vip)" {
            n173 = control-ref of="Publish"() -> (w379:refnum<vi>)
            n174 = property class="Bool"(reference=w379, "DisabledEnum"=T4."Enabled" ("Disabled")) -> ()  [unwired: 1 in, 2 out]
          }
          frame "LV Project (lvproj)" {
          }
          frame "Build Spec (vipb)" {
            n175 = case shown="True" w381 {
              tunnel: w382 -> [_ w383]
              frame False {
              }
              frame True {
                n176 = for {
                  tunnel: w383 -> [w384] mode=indexing
                  n177 = property class="Ctl"(reference=w384, "DisabledEnum"=T4."Enabled" ("Disabled")) -> ()  [unwired: 1 in, 2 out]
                }
              }
            }
          }
        }
        n178 = call <vilib>:"Add State(s) to Queue__jki_lib_state_machine.vi"("State(s) in (\"\")"=w378) -> ("States Out"=w377:string)  [unwired: 14 in]
      }
      frame "UI: Cursor Set" {
        # "Argument"
        # "Set and Unset Cursor Busy.\n(Usage: \"UI: Cursor Set >> Busy|Idle\")"
        n179 = case shown="\"Busy\"" w386 {
          tunnel: w388 -> [w393 w395]
          tunnel: [w392 w394] -> w387
          frame "Idle", Default {
            n180 = call <vilib>:"Unset Busy.vi"("error in (no error)"=w393) -> ("error out"=w392:errorcluster)  [unwired: 10 in]
          }
          frame "Busy" {
            n181 = call <vilib>:"Set Busy.vi"("error in (no error)"=w395) -> ("error out"=w394:errorcluster)  [unwired: 9 in, 1 out]
          }
        }
        n182 = call <vilib>:"Add State(s) to Queue__jki_lib_state_machine.vi"("State(s) in (\"\")"=w391) -> ("States Out"=w390:string)  [unwired: 14 in]
      }
      frame "UI: Front Panel State" {
        # "Argument"
        # "Set Front Panel Open or Closed\n(Usage: \"UI: Front Panel State >> Open|Close\")"
        n183 = Unbundle By Name(w398) -> ("Core.Current VI Reference"=w397:refnum<vi>)
        n184 = case shown="\"Open\", \"Standard\", Default" w396 {
          tunnel: w400 -> [w408 w423 w434 w447 w460]
          tunnel: [w410 w424 w436 w449 w462] -> w399
          tunnel: w397 -> [w409 w421 w435 w448 w461]
          frame "Open", "Standard", Default {
            w403 = T2."Standard" ("State")
            n185 = property class="VI"(reference=w409, error in=w408) -> (reference out=w406:refnum<vi>, error out=w407:errorcluster, "FP.State"=w405:T2)
            n186 = Not Equal?(x=w405, y=w403) -> (x != y?=w404:bool)
            n187 = case shown="False" w404 {
              tunnel: [w414 w416] -> w410
              tunnel: w407 -> [w413 w416]
              tunnel: w406 -> [w412 _]
              tunnel: w403 -> [w411 _]
              frame True {
                n188 = invoke class="VI" method="FP.Open"(reference=w412, error in=w413, "Activate"=TRUE, "State"=w411) -> (error out=w414:errorcluster)  [unwired: 1 in, 4 out]
              }
              frame False {
              }
            }
          }
          frame "Close", "Closed" {
            n189 = property class="VI"(reference=w421, error in=w423) -> (reference out=w420:refnum<vi>, error out=w422:errorcluster, "FP.State"=w418:T2)
            n190 = Not Equal?(x=w418, y=T2."Closed" ("Front Panel Window:State")) -> (x != y?=w417:bool)
            n191 = case shown="True" w417 {
              tunnel: [w425 w428] -> w424
              tunnel: w422 -> [w425 w427]
              tunnel: w420 -> [_ w426]
              frame False {
              }
              frame True {
                n192 = invoke class="VI" method="FP.Close"(reference=w426, error in=w427) -> (error out=w428:errorcluster)  [unwired: 1 in, 2 out]
              }
            }
          }
          frame "Hidden", "Hide" {
            w429 = T2."Hidden" ("State")
            n193 = property class="VI"(reference=w435, error in=w434) -> (reference out=w432:refnum<vi>, error out=w433:errorcluster, "FP.State"=w431:T2)
            n194 = Not Equal?(x=w431, y=w429) -> (x != y?=w430:bool)
            n195 = case shown="True" w430 {
              tunnel: [w440 w441] -> w436
              tunnel: w433 -> [w439 w441]
              tunnel: w432 -> [w438 _]
              tunnel: w429 -> [w437 _]
              frame True {
                n196 = invoke class="VI" method="FP.Open"(reference=w438, error in=w439, "State"=w437) -> (error out=w440:errorcluster)  [unwired: 2 in, 4 out]
              }
              frame False {
              }
            }
          }
          frame "Minimize", "Minimized" {
            w442 = T2."Minimized" ("State")
            n197 = property class="VI"(reference=w448, error in=w447) -> (reference out=w445:refnum<vi>, error out=w446:errorcluster, "FP.State"=w444:T2)
            n198 = Not Equal?(x=w444, y=w442) -> (x != y?=w443:bool)
            n199 = case shown="True" w443 {
              tunnel: [w453 w454] -> w449
              tunnel: w446 -> [w452 w454]
              tunnel: w445 -> [w451 _]
              tunnel: w442 -> [w450 _]
              frame True {
                n200 = invoke class="VI" method="FP.Open"(reference=w451, error in=w452, "State"=w450) -> (error out=w453:errorcluster)  [unwired: 2 in, 4 out]
              }
              frame False {
              }
            }
          }
          frame "Maximize", "Maximized" {
            w455 = T2."Maximized" ("State")
            n201 = property class="VI"(reference=w461, error in=w460) -> (reference out=w458:refnum<vi>, error out=w459:errorcluster, "FP.State"=w457:T2)
            n202 = Not Equal?(x=w457, y=w455) -> (x != y?=w456:bool)
            n203 = case shown="True" w456 {
              tunnel: [w466 w467] -> w462
              tunnel: w459 -> [w465 w467]
              tunnel: w458 -> [w464 _]
              tunnel: w455 -> [w463 _]
              frame True {
                n204 = invoke class="VI" method="FP.Open"(reference=w464, error in=w465, "State"=w463) -> (error out=w466:errorcluster)  [unwired: 2 in, 4 out]
              }
              frame False {
              }
            }
          }
        }
        n205 = call <vilib>:"Add State(s) to Queue__jki_lib_state_machine.vi"("State(s) in (\"\")"=w402) -> ("States Out"=w401:string)  [unwired: 14 in]
      }
      frame "---------- Macro ----------" {
        # "Do not put any code in this frame.\n(It is a separator no-op. You can make a copy of this frame to create a new Macro frame)"
        n206 = call <vilib>:"Add State(s) to Queue__jki_lib_state_machine.vi"("State(s) in (\"\")"=w471) -> ("States Out"=w470:string)  [unwired: 14 in]
      }
      frame "Macro: Initialize" {
        w472 = "Data: Initialize\nInitialize Core Data\nUI: Initialize\nUI: Front Panel State >> Open\n\nMacro: Read File"  # Data: Initialize Initialize Core Data UI: Initialize UI: Front Panel State >> Open  Macro: Read File
        # "Initialization Macro\n(This is called once, when the VI starts)"
        n207 = call <vilib>:"Add State(s) to Queue__jki_lib_state_machine.vi"("State(s) in Front (\"\")"=w472, "State(s) in (\"\")"=w476) -> ("States Out"=w475:string)  [unwired: 13 in]
      }
      frame "Macro: Read File" {
        # "Initialization Macro\n(This is called once, when the VI starts)"
        n208 = call <vilib>:"Add State(s) to Queue__jki_lib_state_machine.vi"("State(s) in Front (\"\")"="UI: Cursor Set >> Busy\nUI: Disable Buttons\nData: Choose File List\nData: Read File List\nData: Update Listbox\nUI: Enable Buttons\nUI: Cursor Set >> Idle", "State(s) in (\"\")"=w481) -> ("States Out"=w480:string)  [unwired: 13 in]
      }
      frame "Macro: Exit" {
        # "Exit Macro\n(This is called once, when the VI exits)"
        n209 = Unbundle By Name(w488) -> ("Core.Close Panel on Exit?"=w487:bool)
        n210 = Select(t="UI: Front Panel State >> Close", s=w487, f="") -> (s? t:f=w484:string)
        n211 = call <vilib>:"Add State(s) to Queue__jki_lib_state_machine.vi"("State(s) in (\"\")"=w484, "State(s) at Back (\"\")"="Data: Cleanup\nExit") -> ("States Out"=w482:string)  [unwired: 13 in]
        n212 = call <vilib>:"Add State(s) to Queue__jki_lib_state_machine.vi"("State(s) in Front (\"\")"=w482, "State(s) in (\"\")"=w491) -> ("States Out"=w490:string)  [unwired: 13 in]
      }
      frame "---------- Action ----------" {
        # "Template Separator\n(You can make a copy of, or modify, this frame)"
        n213 = call <vilib>:"Add State(s) to Queue__jki_lib_state_machine.vi"("State(s) in (\"\")"=w495) -> ("States Out"=w494:string)  [unwired: 14 in]
      }
      frame "Action: Open File" {
        # "Your code here.\n(You can make a copy of, or modify, this frame)"
        n214 = Unbundle By Name(w506) -> ("selected path"=w496:path)
        n215 = Format Into String(format string="cmd /c explorer.exe \"%s\"", error in=w500, w496) -> (resulting string=w504:string, error out=w502:errorcluster)  [unwired: 1 in]
        n216 = Strip Path(path=w496) -> (name=w498:string)  [unwired: 1 out]
        n217 = call <vilib>:"System Exec.vi"("run minimized? (F)"=TRUE, "error in (no error)"=w502, "command line"=w504) -> ("error out"=w501:errorcluster)  [unwired: 5 in, 3 out]
        n218 = Format Into String(format string="Opening \"%s\"...", w498) -> (resulting string=w499:string)  [unwired: 2 in, 1 out]
        n219 = local write "Status"(w499) -> ()
        n220 = call <vilib>:"Add State(s) to Queue__jki_lib_state_machine.vi"("State(s) in (\"\")"=w508) -> ("States Out"=w507:string)  [unwired: 14 in]
      }
      frame "---------- VIPM ----------" {
        # "Template Separator\n(You can make a copy of, or modify, this frame)"
        n221 = call <vilib>:"Add State(s) to Queue__jki_lib_state_machine.vi"("State(s) in (\"\")"=w512) -> ("States Out"=w511:string)  [unwired: 14 in]
      }
      frame "VIPM: Preview VIPB" {
        # "Your code here.\n(You can make a copy of, or modify, this frame)"
        n222 = Unbundle By Name(w523) -> ("vipb paths"=w519:path[], "selected path"=w521:path)
        n223 = local read "ALL"() -> (w517:bool)
        n224 = Build Array(w521) -> (w518:path[])
        n225 = Select(t=w519, s=w517, f=w518) -> (s? t:f=w520:path[])
        n226 = for {
          tunnel: w520 -> [w529] mode=indexing
          tunnel: [w532] -> w515
          tunnel: w522 -> [w531]
          tunnel: [w530] -> w516 mode=indexing
          n227 = Strip Path(path=w529) -> (name=w526:string)  [unwired: 1 out]
          n228 = Format Into String(format string="Reading \"%s\"...", w526) -> (resulting string=w528:string)  [unwired: 2 in, 1 out]
          n229 = call <vilib>:"Read VI Package Build Spec_vipm_api.vi"("error in (no error)"=w531, "Path to VIPB File"=w529) -> ("error out"=w532:errorcluster, "VI Package Build Spec Data"=w530:T8)  [unwired: 8 in]
          n230 = local write "Status"(w528) -> ()
        }
        n231 = call "Format Build Spec Summary.vi"("error in (no error)"=w515, "Build Spec [] in"=w516) -> ("error out"=w514:errorcluster, "VIPB Preview"=w513:string)  [unwired: 8 in]
        n232 = local write "Status"(w513) -> ()
        n233 = call <vilib>:"Add State(s) to Queue__jki_lib_state_machine.vi"("State(s) in (\"\")"=w525) -> ("States Out"=w524:string)  [unwired: 14 in]
      }
      frame "VIPM: Increment Patch" {
        # "Your code here.\n(You can make a copy of, or modify, this frame)"
        n234 = Unbundle By Name(w543) -> ("vipb paths"=w540:path[], "selected path"=w542:path)
        n235 = local read "ALL"() -> (w537:bool)
        n236 = Build Array(w542) -> (w539:path[])
        n237 = Select(t=w540, s=w537, f=w539) -> (s? t:f=w541:path[])
        n238 = for {
          tunnel: w541 -> [w547] mode=indexing
          tunnel: w538 -> [w552]
          tunnel: [w548] -> w536
          tunnel: [w546] -> w534 mode=indexing
          n239 = Strip Path(path=w547) -> (name=w549:string)  [unwired: 1 out]
          n240 = Format Into String(format string="Updating \"%s\"...", w549) -> (resulting string=w551:string)  [unwired: 2 in, 1 out]
          n241 = call "Increment Patch.vi"("error in (no error)"=w552, "selected path"=w547) -> ("error out"=w548:errorcluster, "VI Package Build Spec Data"=w546:T8)  [unwired: 8 in]
          n242 = local write "Status"(w551) -> ()
        }
        n243 = call "Format Build Spec Summary.vi"("error in (no error)"=w536, "Build Spec [] in"=w534) -> ("error out"=w535:errorcluster, "VIPB Preview"=w533:string)  [unwired: 8 in]
        n244 = local write "Status"(w533) -> ()
        n245 = call <vilib>:"Add State(s) to Queue__jki_lib_state_machine.vi"("State(s) in (\"\")"=w545) -> ("States Out"=w544:string)  [unwired: 14 in]
      }
      frame "VIPM: Clear Notes" {
        # "Your code here.\n(You can make a copy of, or modify, this frame)"
        n246 = Unbundle By Name(w563) -> ("vipb paths"=w560:path[], "selected path"=w562:path)
        n247 = local read "ALL"() -> (w557:bool)
        n248 = Build Array(w562) -> (w559:path[])
        n249 = Select(t=w560, s=w557, f=w559) -> (s? t:f=w561:path[])
        n250 = for {
          tunnel: w561 -> [w566] mode=indexing
          tunnel: w558 -> [w572]
          tunnel: [w567] -> w556 mode=indexing
          tunnel: [w568] -> w555
          n251 = Strip Path(path=w566) -> (name=w569:string)  [unwired: 1 out]
          n252 = Format Into String(format string="Updating \"%s\"...", w569) -> (resulting string=w571:string)  [unwired: 2 in, 1 out]
          n253 = call "Clear Change Log.vi"("error in (no error)"=w572, "selected path"=w566) -> ("error out"=w568:errorcluster, "VI Package Build Spec Data"=w567:T8)  [unwired: 8 in]
          n254 = local write "Status"(w571) -> ()
        }
        n255 = call "Format Build Spec Summary.vi"("error in (no error)"=w555, "Build Spec [] in"=w556) -> ("error out"=w554:errorcluster, "VIPB Preview"=w553:string)  [unwired: 8 in]
        n256 = local write "Status"(w553) -> ()
        n257 = call <vilib>:"Add State(s) to Queue__jki_lib_state_machine.vi"("State(s) in (\"\")"=w565) -> ("States Out"=w564:string)  [unwired: 14 in]
      }
      frame "VIPM: Append Notes" {
        # "Your code here.\n(You can make a copy of, or modify, this frame)"
        n258 = Unbundle By Name(w582) -> ("vipb paths"=w579:path[], "selected path"=w581:path)
        n259 = local read "ALL"() -> (w576:bool)
        n260 = Build Array(w581) -> (w578:path[])
        n261 = Select(t=w579, s=w576, f=w578) -> (s? t:f=w580:path[])
        n262 = for {
          tunnel: w580 -> [w585] mode=indexing
          tunnel: w577 -> [w592]
          tunnel: [w588] -> w575
          tunnel: [w587] -> w574 mode=indexing
          n263 = Strip Path(path=w585) -> (name=w589:string)  [unwired: 1 out]
          n264 = Format Into String(format string="Updating \"%s\"...", w589) -> (resulting string=w591:string)  [unwired: 2 in, 1 out]
          n265 = call "Append to Change Log.vi"("error in (no error)"=w592, "Release Notes"="Release Notes", "selected path"=w585) -> ("error out"=w588:errorcluster, "VI Package Build Spec Data"=w587:T8)  [unwired: 7 in]
          n266 = local write "Status"(w591) -> ()
        }
        n267 = call "Format Build Spec Summary.vi"("Build Spec [] in"=w574) -> ("VIPB Preview"=w573:string)  [unwired: 9 in, 1 out]
        n268 = local write "Status"(w573) -> ()
        n269 = call <vilib>:"Add State(s) to Queue__jki_lib_state_machine.vi"("State(s) in (\"\")"=w584) -> ("States Out"=w583:string)  [unwired: 14 in]
      }
      frame "VIPM: Build" {
        # "Template Separator\n(You can make a copy of, or modify, this frame)"
        n270 = Unbundle By Name(w603) -> ("vipb paths"=w606:path[], "selected path"=w608:path)
        n271 = local read "ALL"() -> (w600:bool)
        n272 = Build Array(w608) -> (w605:path[])
        n273 = Select(t=w606, s=w600, f=w605) -> (s? t:f=w607:path[])
        n274 = for {
          tunnel: w607 -> [w623] mode=indexing
          tunnel: [w628] -> w602 mode=indexing
          tunnel: w596 -> [w621]
          tunnel: [w626] -> w595 mode=indexing
          n275 = call "Message.vi"("Status"="Git Flow Release Start" ("format string"), "error in (no error)"=w621, "selected path"=w623) -> ("error out"=w622:errorcluster, "selected path out"=w618:path, "Message out"=w624:string)  [unwired: 6 in]
          n276 = local write "Status"(w624) -> ()
          n277 = call "Macro Start Release.vi"("error in (no error)"=w622, "VIPB Path"=w618) -> ("error out"=w620:errorcluster, "Git out"=w627:refnum<class "Git.lvclass">)  [unwired: 8 in]
          n278 = call "Message.vi"("Status"="VIPM Building" ("format string"), "error in (no error)"=w620, "selected path"=w618) -> ("error out"=w619:errorcluster, "selected path out"=w616:path, "Message out"=w617:string)  [unwired: 6 in]
          n279 = local write "Status"(w617) -> ()
          n280 = call <vilib>:"Build VI Package_vipm_api.vi"("error in (no error)"=w619, "Path to VIPB File"=w616) -> ("error out"=w614:errorcluster, "Build Output"=w628:path)  [unwired: 8 in]
          n281 = call "Message.vi"("Status"="Git Flow Release Finish" ("format string"), "error in (no error)"=w614, "selected path"=w616) -> ("error out"=w615:errorcluster, "Message out"=w611:string)  [unwired: 6 in, 1 out]
          n282 = local write "Status"(w611) -> ()
          n283 = call "Macro Finish Release.vi"("error in (no error)"=w615, "Git in"=w627) -> ("error out"=w626:errorcluster)  [unwired: 8 in, 1 out]
        }
        n284 = call <vilib>:"Build State String with Arguments__JKI_lib_State_Machine.vi"("Arguments (\"\")"=w598, "State"="VIPM: Preview VIPB" ("State(s) in Front (\"\")")) -> ("State with Arguments"=w601:string)  [unwired: 4 in]
        n285 = Bundle By Name(cluster=w603, "vip paths"=w602) -> (w604:T5)
        n286 = Merge Errors(w595) -> (w594:errorcluster)
        n287 = property on="Mode" class="Enum (strict)"(error in=w594, "Val(Sgnl)"=File_Type--enum."Package (vip)" ("Value (Signaling)")) -> ()  [unwired: 1 in, 2 out]
        n288 = call <vilib>:"Add State(s) to Queue__jki_lib_state_machine.vi"("State(s) in Front (\"\")"=w601, "State(s) in (\"\")"=w610, "State(s) at Back (\"\")"="Data: Update Listbox" ("State(s) at Back (\"\")")) -> ("States Out"=w609:string)  [unwired: 12 in]
      }
      frame "VIPM: Publish" {
        # "Template Separator\n(You can make a copy of, or modify, this frame)"
        n289 = Unbundle By Name(w636) -> ("vip paths"=w635:path[])
        n290 = call <vilib>:"List VIPM Managed Repositories_vipm_api.vi"("error in (no error)"=w633) -> ("Managed Repositories Info"=w637:T10[], "error out"=w638:errorcluster)  [unwired: 13 in]
        n291 = Index Array(array=w637) -> (element=w639:T10)  [unwired: 1 in]
        n292 = Unbundle By Name(w639) -> ("Repository Name"=w640:string)
        n293 = call <vilib>:"Publish VI Packages to Repository_vipm_api.vi"("error in (no error)"=w638, "Repository Name"=w640, "Packages to publish to Repository Library (vip,ogp)"=w635) -> ("error out"=w634:errorcluster, "Package Names Published"=w630:string[])  [unwired: 7 in]
        n294 = Build Array (concatenate)("Packages Published:", w630) -> (w629:string[])
        n295 = call <vilib>:"1D String Array to Delimited String.vi"("delimiter"="\n", "string array"=w629) -> ()  [unwired: 9 in, 1 out]
        n296 = call <vilib>:"Add State(s) to Queue__jki_lib_state_machine.vi"("State(s) in (\"\")"=w642) -> ("States Out"=w641:string)  [unwired: 14 in]
      }
      frame "---------- git ----------" {
        # "Template Separator\n(You can make a copy of, or modify, this frame)"
        n297 = call <vilib>:"Add State(s) to Queue__jki_lib_state_machine.vi"("State(s) in (\"\")"=w646) -> ("States Out"=w645:string)  [unwired: 14 in]
      }
      frame "git: Execute git flow" {
        # "Your code here.\n(You can make a copy of, or modify, this frame)"
        n298 = Unbundle By Name(w649) -> ("vip paths"=w647:path[])  [unwired: 1 out]
        n299 = for {
          tunnel: w647 -> [w656] mode=indexing
          # "starting at builds\\latest\\*.vip"
          n300 = call "Walk Up to Repository.vi"("Build Path"=w656) -> ("Repository Path"=w655:path)  [unwired: 9 in, 1 out]
          "repository path" <- w655
          n301 = call "Walk Down to Latest Build.vi"("Repository Path"=w655) -> ("Latest Build Folder"=w654:path)  [unwired: 9 in, 1 out]
          n302 = call <vilib>:"Recursive File List.vi"("pattern"="*.vip", "Folder Path"=w654) -> ("error out"=w661:errorcluster, "All Files in Dir"=w660:path[], "dup Folder Path"=w659:path)  [unwired: 5 in, 2 out]
          n303 = call "Find Most Recent File.vi"("error in (no error)"=w661, "All Files in Dir"=w660) -> ("error out"=w662:errorcluster, "Path"=w653:path)  [unwired: 8 in]
          "Latest VIP" <- w653
          n304 = call <vilib>:"Recursive File List.vi"("pattern"="*.exe", "error in (no error)"=w662, "Folder Path"=w659) -> ("error out"=w664:errorcluster, "All Files in Dir"=w663:path[])  [unwired: 4 in, 3 out]
          n305 = call "Find Most Recent File.vi"("error in (no error)"=w664, "All Files in Dir"=w663) -> ("Path"=w652:path)  [unwired: 8 in, 1 out]
          "Latest EXE" <- w652
          n306 = Build Array(w653, w652) -> ()  [unwired: 1 out]
        }
        n307 = call <vilib>:"Add State(s) to Queue__jki_lib_state_machine.vi"("State(s) in (\"\")"=w651) -> ("States Out"=w650:string)  [unwired: 14 in]
      }
    }
  }
  n308 = disable-structure shown="Disabled" {
    frame Disabled {
      n309 = call <vilib>:"Read VI Package Build Spec_vipm_api.vi"() -> ("VI Package Build Spec Data"=w670:T8)  [unwired: 10 in, 1 out]
      n310 = Unbundle By Name(w670) -> ("Package Version.major"=w668:u32, "Package Version.minor"=w667:u32, "Package Version.patch"=w666:u32, "Package Version.build"=w665:u32)
      n311 = Format Into String(format string="v%d.%d.%d.%d", w668, w667, w666, w665) -> ()  [unwired: 2 in, 2 out]
    }
    frame Enabled {
    }
  }
